vi "KHETS - Config Instruments.vi"(8 "Instrument Locations In":T2, 11 "Instruments In":T7={"Magnet"=enum."Manual", "Ammeter"=enum."648X", "Current Source"=enum."622X", "Switch"=enum."3706A", "Voltmeter"=enum."2182A"}) -> (0 "Instrument Locations Out":T2, 2 "Clicked OK?":bool, 3 "Instruments Out":T7={"Magnet"=enum."Manual", "Ammeter"=enum."648X", "Current Source"=enum."622X", "Switch"=enum."3706A", "Voltmeter"=enum."2182A"})   [LabVIEW 2018]
uses:
  <instrlib>/Hall Effect Library/Public/Controls/Ammeters.ctl
  <instrlib>/Hall Effect Library/Public/Controls/I-Sources.ctl
  <instrlib>/Hall Effect Library/Public/Controls/Switches.ctl
  <instrlib>/Hall Effect Library/Public/Controls/Voltmeters.ctl
  <instrlib>/Hall Effect Library/Public/Controls/Magnets.ctl
  <instrlib>/Hall Effect Library/Hall Effect Library.lvlib
panel:
  in  "Magnet Location":refnum<visa-resource-name>
  in  "Magnet":T1
  in  "cmdCancel":bool
  in  "cmdOK":bool
  in  "Voltmeter Location":refnum<visa-resource-name>
  in  "Switch Location":refnum<visa-resource-name>
  in  "Current Source Location":refnum<visa-resource-name>
  in  "Ammeter Location":refnum<visa-resource-name>
  in  "Voltmeter":T6=enum."2182A"
  in  "Switch":T5
  in  "Current Source":T4
  in  "Ammeter":T3=enum."648X"
  # "Configure Instruments"
  # "Model"
  # "Location"
  # "Magnet"
  # "Ammeter"
  # "Current Source"
  # "Switch"
  # "Voltmeter"
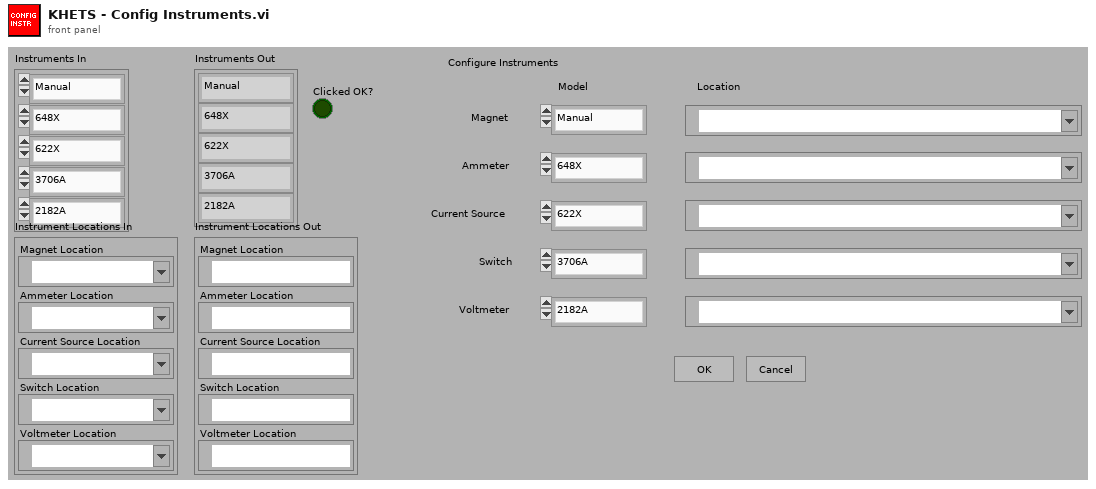
[diagram p1: front panel]
types:
  T1 = typedef "Hall Effect Library.lvlib/Magnets.ctl" = enum16{"Manual"}
  T2 = cluster{"Magnet Location":refnum<visa-resource-name>, "Ammeter Location":refnum<visa-resource-name>, "Current Source Location":refnum<visa-resource-name>, "Switch Location":refnum<visa-resource-name>, "Voltmeter Location":refnum<visa-resource-name>}
  T3 = typedef "Hall Effect Library.lvlib/Ammeters.ctl" = enum16{"None", "648X"}
  T4 = typedef "Hall Effect Library.lvlib/I-Sources.ctl" = enum16{"622X", "26XX"}
  T5 = typedef "Hall Effect Library.lvlib/Switches.ctl" = enum16{"3706A"}
  T6 = typedef "Hall Effect Library.lvlib/Voltmeters.ctl" = enum16{"2000", "2182A", "3706A"}
  T7 = cluster{"Magnet":T1, "Ammeter":T3, "Current Source":T4, "Switch":T5, "Voltmeter":T6}
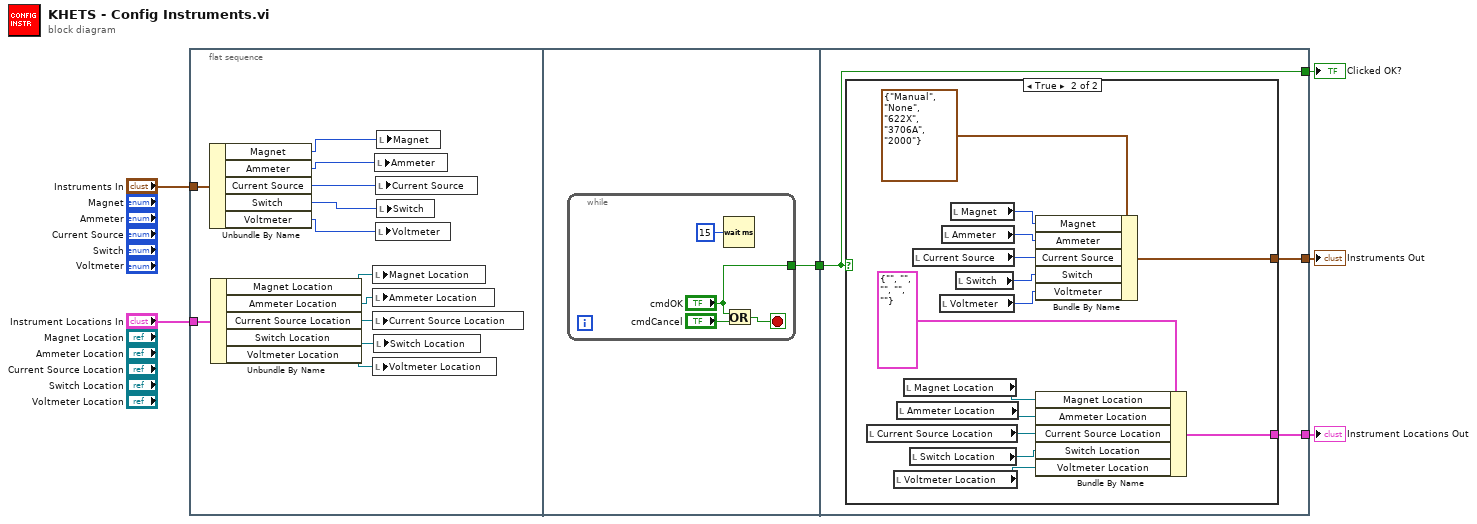
[diagram p0: block diagram]
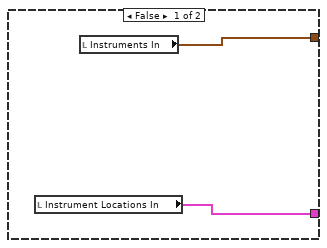
[diagram p2: hidden frame]
diagram:
  n1 = flat-sequence {
    tunnel: "Instruments In" -> [w18]
    tunnel: "Instrument Locations In" -> [w17]
    tunnel: [w19] -> w4
    tunnel: w4 -> [w24]
    tunnel: [w26] -> w3
    tunnel: [w25] -> w2
    tunnel: [w24] -> w1
    frame #0 {
      n2 = Unbundle By Name(w18) -> ("Magnet"=w7:T1, "Ammeter"=w10:T3, "Current Source"=w11:T4, "Switch"=w12:T5, "Voltmeter"=w9:T6)
      n3 = Unbundle By Name(w17) -> ("Magnet Location"=w8:refnum<visa-resource-name>, "Ammeter Location"=w14:refnum<visa-resource-name>, "Current Source Location"=w15:refnum<visa-resource-name>, "Switch Location"=w16:refnum<visa-resource-name>, "Voltmeter Location"=w13:refnum<visa-resource-name>)
      n4 = local write "Magnet Location"(w8) -> ()
      n5 = local write "Ammeter Location"(w14) -> ()
      n6 = local write "Current Source Location"(w15) -> ()
      n7 = local write "Voltmeter Location"(w13) -> ()
      n8 = local write "Switch Location"(w16) -> ()
      n9 = local write "Ammeter"(w10) -> ()
      n10 = local write "Current Source"(w11) -> ()
      n11 = local write "Voltmeter"(w9) -> ()
      n12 = local write "Magnet"(w7) -> ()
      n13 = local write "Switch"(w12) -> ()
    }
    frame #1 {
      n14 = while {
        tunnel: ["cmdOK"] -> w19
        stop <- w23 stop-if-true
        n15 = Wait (ms)(milliseconds to wait=u32 15) -> ()  [unwired: 1 out]
        n16 = Or(x="cmdOK", y="cmdCancel") -> (x .or. y?=w23:bool)
      }
    }
    frame #2 {
      n17 = case shown="True" w24 {
        tunnel: [w28 w34] -> w26
        tunnel: [w27 w29] -> w25
        frame False {
          n18 = local read "Instrument Locations In"() -> (w27:T2)
          n19 = local read "Instruments In"() -> (w28:T7)
        }
        frame True {
          n20 = local read "Current Source Location"() -> (w42:refnum<visa-resource-name>)
          n21 = local read "Voltmeter Location"() -> (w39:refnum<visa-resource-name>)
          n22 = local read "Ammeter Location"() -> (w40:refnum<visa-resource-name>)
          n23 = local read "Magnet Location"() -> (w30:refnum<visa-resource-name>)
          n24 = local read "Switch Location"() -> (w41:refnum<visa-resource-name>)
          n25 = local read "Current Source"() -> (w38:T4)
          n26 = local read "Voltmeter"() -> (w35:T6)
          n27 = local read "Ammeter"() -> (w36:T3)
          n28 = local read "Magnet"() -> (w32:T1)
          n29 = local read "Switch"() -> (w37:T5)
          n30 = Bundle By Name(cluster=T7 {"Magnet"=enum."Manual", "Ammeter"=enum."None", "Current Source"=enum."622X", "Switch"=enum."3706A", "Voltmeter"=enum."2000"} ("Instruments In"), "Magnet"=w32, "Ammeter"=w36, "Current Source"=w38, "Switch"=w37, "Voltmeter"=w35) -> (w34:T7)
          n31 = Bundle By Name(cluster=T2 {"Magnet Location"="", "Ammeter Location"="", "Current Source Location"="", "Switch Location"="", "Voltmeter Location"=""} ("Instrument Locations In"), "Magnet Location"=w30, "Ammeter Location"=w40, "Current Source Location"=w42, "Switch Location"=w41, "Voltmeter Location"=w39) -> (w29:T2)
        }
      }
    }
  }
  "Instruments Out" <- w3
  "Instrument Locations Out" <- w2
  "Clicked OK?" <- w1
